vi "DebugLogger.vi"(8 "error in (no error)":errorcluster, 10 "Message":string, 11 "Path":path) -> (0 "error out":errorcluster)   [LabVIEW 2026]
doc: "Diagnostic scaffolding (remove before commit). Appends a tick-stamped line to a fixed debug text file, opening/appending/closing per call so the line commits immediately and survives the actor context. Transparent to the error chain: error in passes to error out unchanged, and the debug write runs regardless of error in. Not part of the library."
uses:
  <vilib>/Utility/miscctls.llb/LVPointTypeDef.ctl
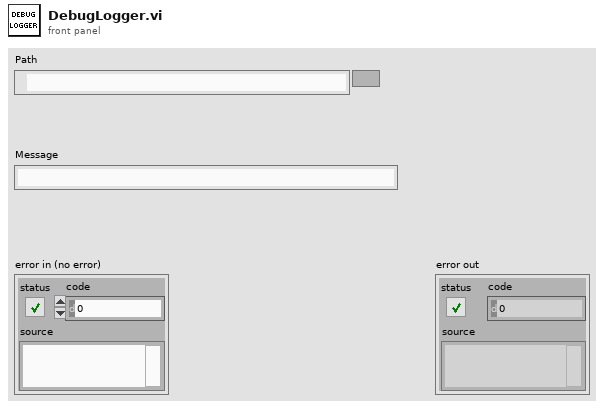
[diagram p1: front panel]
types:
  T1 = typedef "LVPointTypeDef.ctl" = cluster{"Horizontal":i16, "Vertical":i16}
  T2 = enum16{"open", "replace", "create", "open or create", "replace or create", "replace or create with confirmation"}
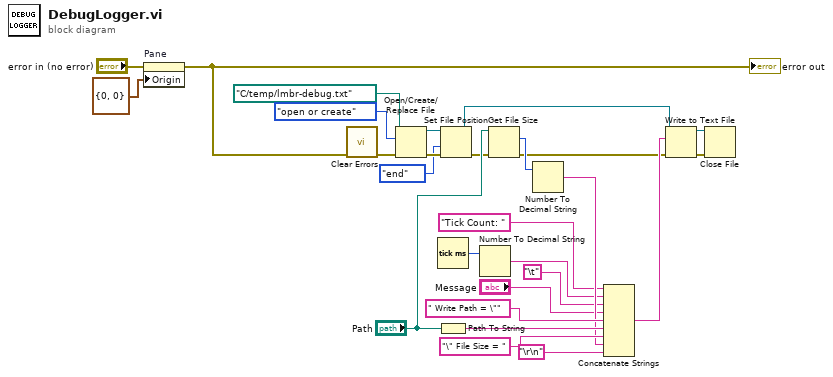
[diagram p0: block diagram]
diagram:
  n1 = property on="Pane" class="Pane"(error in="error in (no error)", "Origin"=T1 {"Horizontal"=0, "Vertical"=0}) -> (error out=w2:errorcluster)  [unwired: 1 in, 1 out]
  "error out" <- w2
  n2 = call <vilib>:"Clear Errors.vi"("error in (no error)"=w2) -> ("error out"=w1:errorcluster)  [unwired: 5 in, 1 out]
  n3 = Open/Create/Replace File(file path (use dialog)=path "C:/temp/lmbr-debug.txt", error in=w1, operation (0:open)=T2."open or create") -> (refnum out=w25:refnum<file>, error out=w24:errorcluster)  [unwired: 3 in, 1 out]
  n4 = Tick Count (ms)() -> (millisecond timer value=w18:u32)
  n5 = Path To String(path="Path") -> (string=w14:string)
  n6 = Set File Position(refnum=w25, from (0:start)=enum16{"start", "end", "current"}."end", error in=w24) -> (refnum out=w22:refnum<file>, error out=w9:errorcluster)  [unwired: 1 in]
  n7 = Number To Decimal String(number=w18) -> (decimal integer string=w5:string)  [unwired: 1 in]
  n8 = Get File Size(file="Path", error in=w9) -> (size (in bytes)=w12:i64, 0:w8:errorcluster)  [unwired: 1 out]
  n9 = Number To Decimal String(number=w12) -> (decimal integer string=w11:string)  [unwired: 1 in]
  n10 = Concatenate Strings("Tick Count: ", w5, "\t", "Message", " Write Path = \"" ("string"), w14, "\" File Size = " ("string"), w11, "\r\n") -> (w21:string)
  n11 = Write to Text File(file (use dialog)=w22, text=w21, error in=w8) -> (refnum out=w19:refnum<file>, error out=w20:errorcluster)  [unwired: 1 in, 1 out]
  n12 = Close File(refnum=w19, error in=w20) -> ()  [unwired: 2 out]
